vi "Add Array of Variant to JSON Object.vi"(7 "Treatment of Infinity/NaN":T1, 8 "error in (no error)":errorcluster, 10 "Array of Variants (with names)":variant[](array[variant]), 11 "JSON Object in":refnum<class "JSON Object.lvclass">) -> (0 "error out":errorcluster, 3 "JSON Object with items added":refnum<class "JSON Object.lvclass">)   [LabVIEW 2020, in "Library Commun.lvlib" / "Variant JSON.lvlib"]
doc: "Adds an array of Variants into a JSON object. Variant data name will be used as the item name (unnamed data is ignored). Clusters are converted to JSON objects. Variants, if empty (void), are converted to null, unless they have attributes, in which case these are converted into a JSON object. \n\nTreatment of Infinity, -Infinity, and Not-a-Number values of floating-point numerics:\n<b>-- Default JSON:</b> write all as nulls.\n<b>-- Extended:</b> use JSON strings for Infinities (\"Infinity\", \"-Infinity\"); NaN still null.\n<b>-- LabVIEW extentions</b> (compatable with the LabVIEW JSON primatives): Infinity, -Infinity, NaN (not in quotes)\n\nNote that the LabVIEW extentions are not valid JSON. The Extended option <b>is</b> valid JSON, but not all JSON parsers will process strings as numeric values.\n\nMore information on http://lavag.org/topic/16217-cr-json-labview"
uses:
  Variant JSON.lvlib
  JSON Object/JSON Object.lvclass
  JSON Scalar/Infinity&NaN.ctl
  support/JSON support.lvlib
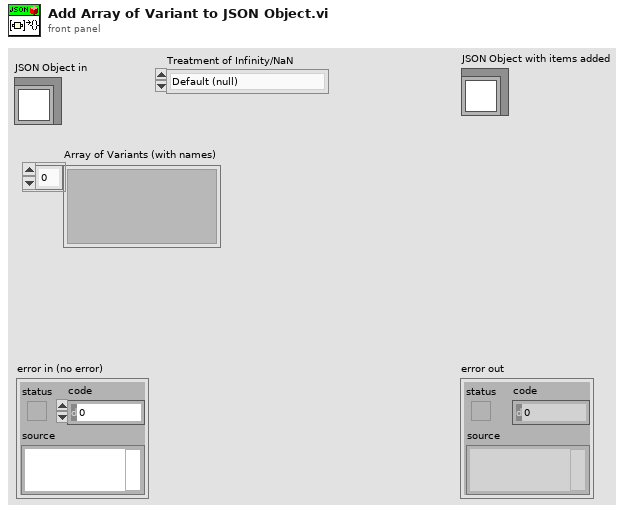
[diagram p1: front panel]
types:
  T1 = typedef "Library Commun.lvlib/JSON support.lvlib/Infinity&NaN.ctl" = enum16{"Default (null)", "Extended", "LabVIEW extensions"}
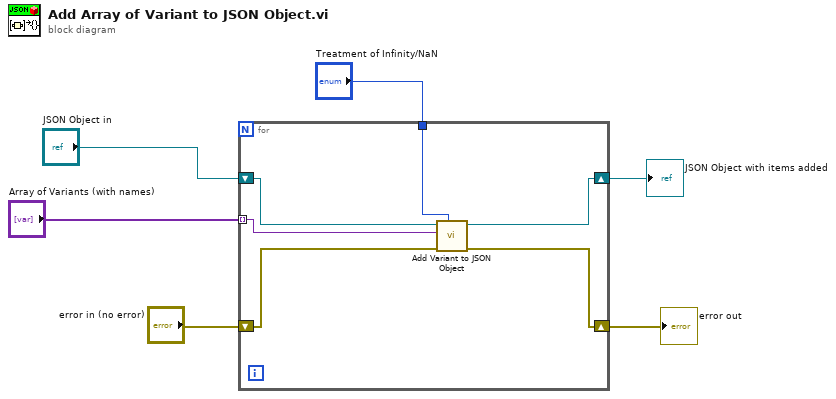
[diagram p0: block diagram]
diagram:
  n1 = for {
    tunnel: "Array of Variants (with names)" -> [w7] mode=indexing
    shift-right: [w11] -> w2
    shift-left: "JSON Object in" -> [w12]
    shift-right: [w9] -> w5
    shift-left: "error in (no error)" -> [w10]
    tunnel: "Treatment of Infinity/NaN" -> [w8]
    n2 = call "Add Variant to JSON Object.vi"("Treatment of Infinity/NaN"=w8, "error in (no error)"=w10, "Variant"=w7, "JSON Object in"=w12) -> ("error out"=w9:errorcluster, "JSON Object out"=w11:refnum<class "JSON Object.lvclass">)  [unwired: 6 in]
  }
  "error out" <- w5
  "JSON Object with items added" <- w2
